vi "UnbundleByName.vi"() -> ()   [LabVIEW 2020]
panel:
  out "Gender":bool
  out "Salary":u32
  out "Age":u8
  out "Name":string
  in  "employee":T1={"Name"="Atul Ghumade", "Age"=29, "Salary"=100000, "Gender"=TRUE}
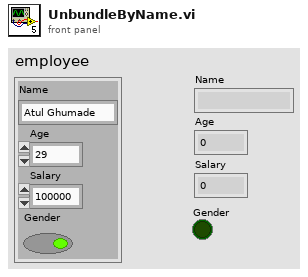
[diagram p1: front panel]
types:
  T1 = cluster{"Name":string, "Age":u8, "Salary":u32, "Gender":bool}
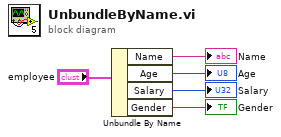
[diagram p0: block diagram]
diagram:
  n1 = Unbundle By Name("employee") -> ("Name"=→"Name":string, "Age"=→"Age":u8, "Salary"=→"Salary":u32, "Gender"=→"Gender":bool)
